vi "RT Loop - Actuation.vi"(8 "error in (no error)":errorcluster, 10 "Actuation Queue":refnum<queue>) -> ()   [LabVIEW 2020]
uses:
  support/Message Queue/Message Cluster.ctl
  controls/FPGA VI Reference.ctl
  Globals/Global - All RT Loop Stop.vi
  <vilib>/rvi/errors/niLvFpgaAdjustHostInterfaceError.vi
  <vilib>/rvi/interface/nirviReadWriteControl/nirviReadWriteControl.xnode
  FPGA Bitfiles/forthexerciseemc_FPGATarget2_FPGAMain_eC4Nf+bThbM.lvbitx
  FPGA Main.vi
  support/Message Queue/Message Queue.lvlib
  NiFpgaLv.dll
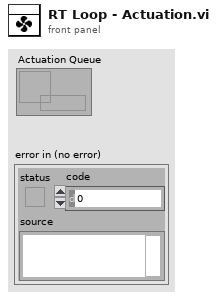
[diagram p1: front panel]
types:
  T1 = typedef "FPGA VI Reference.ctl" = refnum<k20>
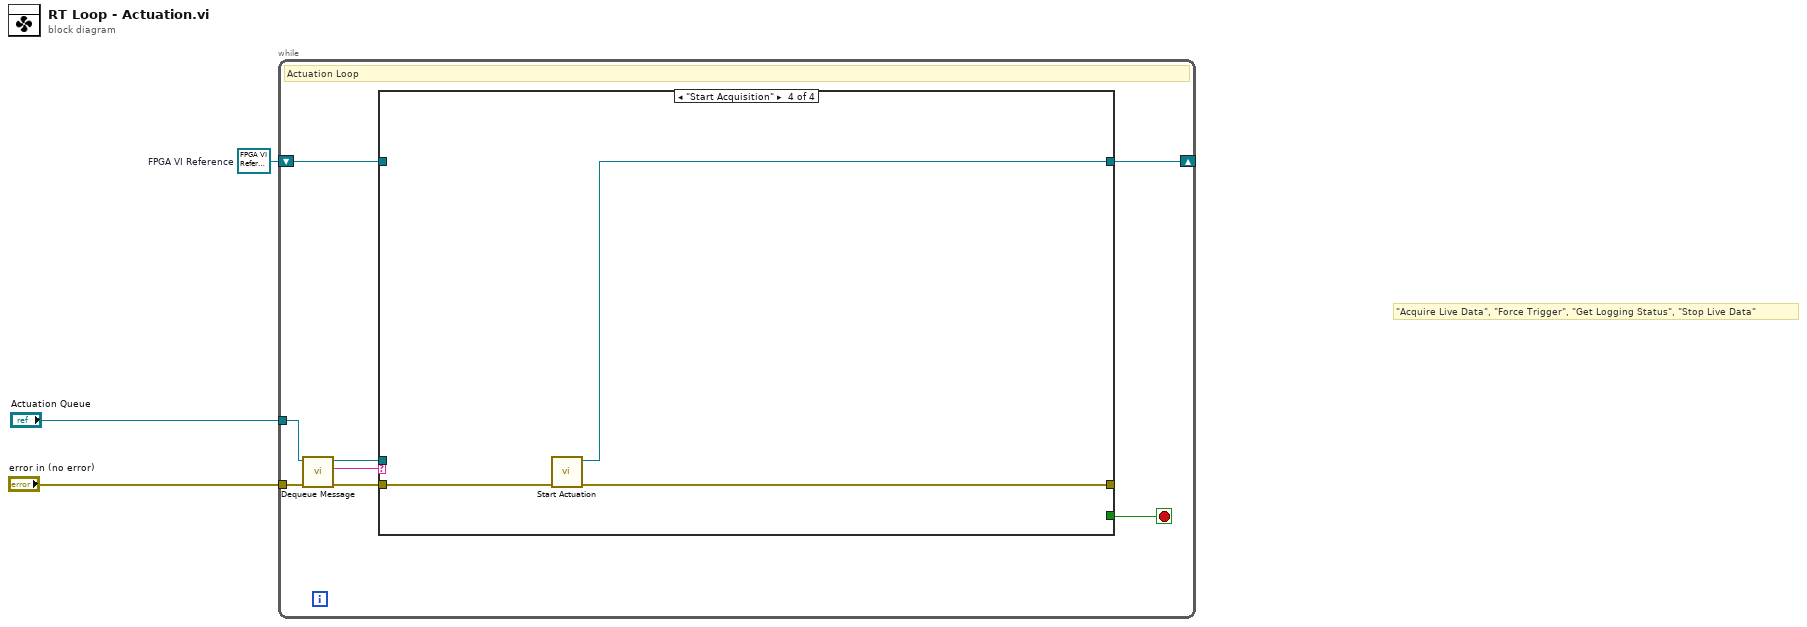
[diagram p0: block diagram]
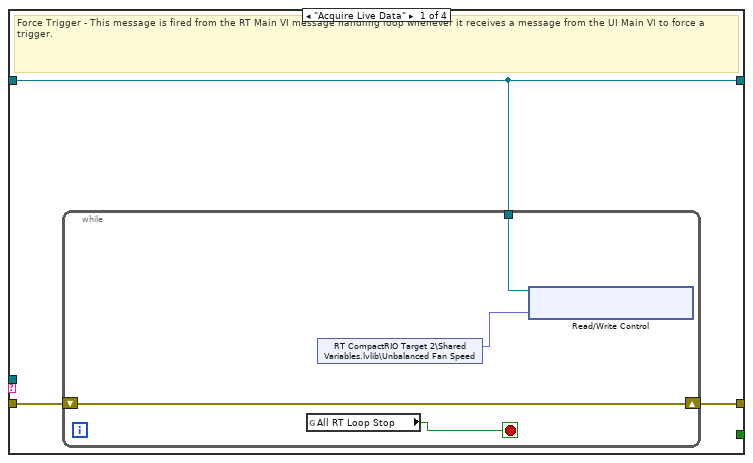
[diagram p2: hidden frame]
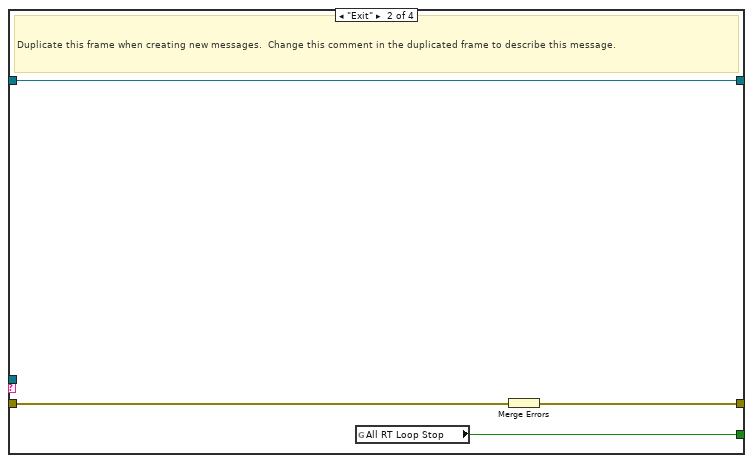
[diagram p3: hidden frame]
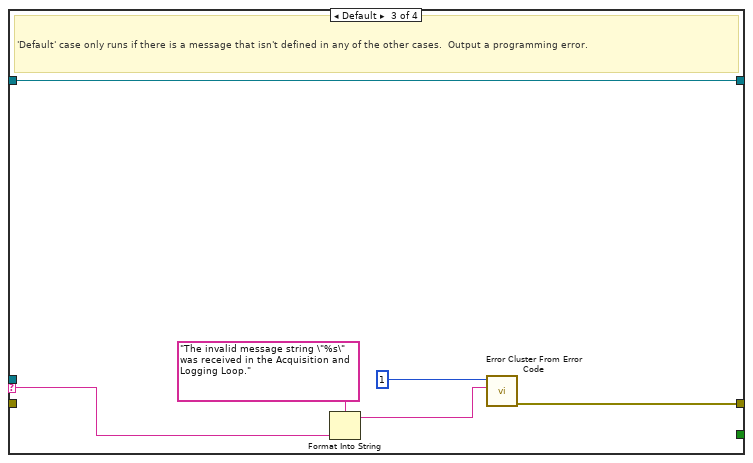
[diagram p4: hidden frame]
diagram:
  w3 = T1 refnum  # FPGA VI Reference
  # "\"Acquire Live Data\", \"Force Trigger\", \"Get Logging Status\", \"Stop Live Data\""
  n1 = while {
    shift-right: [w7] -> _
    shift-left: w3 -> [w8]
    tunnel: "error in (no error)" -> [w6]
    tunnel: "Actuation Queue" -> [w4]
    stop <- w5 stop-if-true
    # "Actuation Loop"
    n2 = call "Dequeue Message.vi"("error in (no error)"=w6, "Message Queue"=w4) -> ("error out"=w11:errorcluster, "Message"=w10:string, "dup Message Queue"=w9:refnum<queue>)  [unwired: 6 in, 1 out]
    n3 = case "Message Cases" shown="\"Start Acquisition\"" w10 {
      selector: w10 -> [_ _ w27 _]
      tunnel: w9 -> [_ _ _ _]
      tunnel: w11 -> [w14 w22 _ w31]
      tunnel: [w13 w21 w25 w29] -> _
      tunnel: [_ w19 _ _] -> w5
      tunnel: w8 -> [w12 w20 w23 _]
      tunnel: [w12 w20 w23 w30] -> w7
      frame "Acquire Live Data" {
        # "Force Trigger - This message is fired from the RT Main VI message handling loop whenever it receives a message from the UI Main VI to force a trigger."
        n4 = while {
          shift-right: [w15] -> w13
          shift-left: w14 -> [w15]
          tunnel: w12 -> [w16]
          stop <- w18 stop-if-true
          n5 = global read "Global - All RT Loop Stop.vi" "All RT Loop Stop"() -> (w18:bool)
          n6 = shared-variable "RT CompactRIO Target 2\\Shared Variables.lvlib\\Unbalanced Fan Speed"() -> (w17:fxp<+/-,20,5>)  [unwired: 1 in, 1 out]
          n7 = xnode "Read/Write Control"("FPGA VI Reference In"=w16, "Unbalanced Fan Speed"=w17) -> ()  [unwired: 1 in, 2 out]
        }
      }
      frame "Exit" {
        # "Duplicate this frame when creating new messages.  Change this comment in the duplicated frame to describe this message."
        n8 = global read "Global - All RT Loop Stop.vi" "All RT Loop Stop"() -> (w19:bool)
        n9 = Merge Errors(w22) -> (w21:errorcluster)
      }
      frame Default {
        # "'Default' case only runs if there is a message that isn't defined in any of the other cases.  Output a programming error."
        n10 = Format Into String(format string="The invalid message string \"%s\" was received in the Acquisition and Logging Loop." ("Unknown Message Error Text"), w27) -> (resulting string=w24:string)  [unwired: 2 in, 1 out]
        n11 = call <vilib>:"Error Cluster From Error Code.vi"("error message (\"\")"=w24, "error code (0)"=1) -> ("error out"=w25:errorcluster)  [unwired: 7 in]
      }
      frame "Start Acquisition" {
        n12 = call "Start Actuation.vi"("error in (no error)"=w31) -> ("error out"=w29:errorcluster, "FPGA VI Reference Out"=w30:T1)  [unwired: 9 in]
      }
    }
  }
